vi "GetImageTimeStamp.vi"(11 "Image refnum in":T1) -> (1 "System Time Stamp":timestamp, 3 "Image (duplicate)":T1)   [LabVIEW 2013]
uses:
  <vilib>/vision/Image Controls.llb/IMAQ Image.ctl
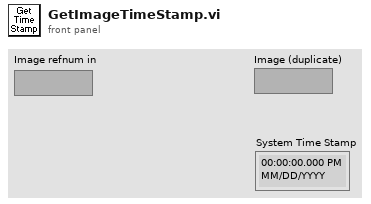
[diagram p1: front panel]
types:
  T1 = typedef "IMAQ Image.ctl" = refnum<image>
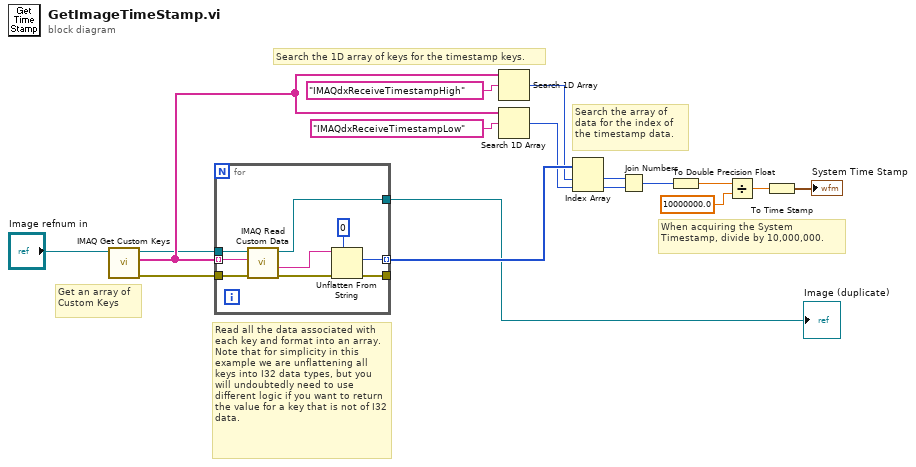
[diagram p0: block diagram]
diagram:
  # "Search the array of data for the index of the timestamp data."
  # "Search the 1D array of keys for the timestamp keys."
  # "Read all the data associated with each key and format into an array. Note that for simplicity in this example we are unflattening all keys into I32 data types, but you will undoubtedly need to use different logic if you want to return the value for a key that is not of I32 data."
  # "Get an array of Custom Keys"
  # "When acquiring the System Timestamp, divide by 10,000,000."
  n1 = call "IMAQ Get Custom Keys"("Image"="Image refnum in") -> ("error out"=w17:errorcluster, "Keys"=w11:string[], "Image (duplicate)"=w3:T1)  [unwired: 7 in, 1 out]
  n2 = for {
    tunnel: w3 -> [w26]
    tunnel: w17 -> [w25]
    tunnel: [w24] -> _
    tunnel: w11 -> [w22] mode=indexing
    tunnel: [w23] -> w1
    tunnel: [w21] -> w16 mode=indexing
    n3 = call "IMAQ Read Custom Data"("error in (no error)"=w25, "Key"=w22, "Image"=w26) -> ("error out"=w20:errorcluster, "Custom Data Out"=w19:string, "Image (duplicate)"=w23:T1)  [unwired: 6 in]
    n4 = Unflatten From String(type=0, binary string=w19, error in (no error)=w20) -> (value=w21:i32, error out=w24:errorcluster)  [unwired: 2 in, 1 out]
  }
  "Image (duplicate)" <- w1
  n5 = Search 1D Array(1D array=w11, element="IMAQdxReceiveTimestampHigh") -> (index of element=w12:i32)  [unwired: 1 in]
  n6 = Search 1D Array(1D array=w11, element="IMAQdxReceiveTimestampLow") -> (index of element=w13:i32)  [unwired: 1 in]
  n7 = Index Array(array=w16, index #1=w12, index #2=w13) -> (element #1=w9:i32, element #2=w10:i32)
  n8 = Join Numbers(hi=w9, lo=w10) -> ((hi.lo)=w8:u64)
  n9 = To Double Precision Float(number=w8) -> (double precision float=w7:dbl)
  n10 = Divide(x=w7, y=10000000.0) -> (x/y=w5:dbl)
  n11 = To Time Stamp(1:w5) -> (0:→"System Time Stamp":timestamp)
